vi "CIS.vi"(2 "Run uninterrupted?":bool, 3 "Device Category IN:":string(combo)="ATLAS18SS" caption="Device Category:", 4 "Batch No.:":string, 5 "Sensor Serial No.:":string, 6 "DB Serial No.:":string) -> (0 "Done!":bool)   [LabVIEW 2019]
doc: "Performs Cis measurements according to ATLAS ITk Quality Control Specifications."
uses:
  general_VIs/globals/QC_MeasurementSetup.vi
  general_VIs/globals/QC_RunInformation.vi
  InstrControl/InstrumentSetup.vi
  InstrControl/Switching/Switching.lvclass
  InstrControl/SupplyControl/SupplyControl.lvclass
  InstrControl/LCRControl/LCRControl.lvclass
  InstrControl/ArduinoControl/ArduinoControl.lvclass
  <vilib>/Analysis/NI_AALBase.lvlib
  InstrControl/InstrControl.lvclass
panel:
  out "Tab Control 2":enum32{"Cis Setup", "Cis Scan"}(tab)
  in  "Current Limit [µA]":dbl=1000.0 min=0.0001 format="%.3f"
  in  "Cis @300V limit [pF/cm]":dbl=1.0
  in  "step interval [s] IN":i32=5 caption="step interval [s]"
  in  "step [V] IN":dbl=10.0 caption="step [V]" format="%.1f"
  in  "Final volts [V] IN":dbl=-500.0 caption="Final volts [V]"
  in  "Initial volts [V] IN":dbl caption="Initial volts [V]"
  in  "Frequency [Hz] Setup":i32=500 caption="Frequency [Hz]" format="%#.3p"
  in  "Measurement Configurations":bool
  in  "Continue":bool
  in  "Quit":bool
  in  "Software current limit?":bool
  out "Capacitance":dbl[](array[numeric]) caption="Cap [pF]"
  out "Volts":dbl[](array[numeric]) caption="Volts [V]"
  out "Resistance":dbl[](array[numeric]) caption="Res [kOhm]"
  out "step interval [s]":u32=5
  out "step [V]":dbl=10.0 format="%.1f"
  out "Final volts [V]":dbl=-700.0 format="%.1f"
  out "Initial volts [V]":dbl format="%.1f"
  out "Frequency [Hz]":i32=100000 format="%#.3p"
  out "RH":dbl[](array[numeric]) caption="RH [%]" format="%#.2f"
  out "Temp.":dbl[](array[numeric]) caption="Temp. [°C]" format="%#.2f"
  out "Cgraph":cluster{"Initial volts":dbl, dbl, dbl[]}(graph)
  in  "Scales":T1(ring)
  in  "Cscale":enum16{"1/C^2 [1/nF^2]", "nF", "pF"}(ring)=enum."pF"
  out "positive ramp?":bool
  out "Tab Control":enum32{"Cis Setup", "Cis Scan"}(tab)
  in  "Switching":string(combo)="Pickering Matrix"
  in  "LCR Meter":string(combo)="WayneKerr 6440B"
  in  "Cis Supply":string(combo)="Keithley 2410"
  in  "Temperature":enum16{"Read Arduino", "Enter manually"}(ring)
  in  "User:":string(combo)="Christoph"
  in  "Hardware Configurations":bool
  in  "Manufacturer:":string(combo)="Hamamatsu"
  in  "abort":bool
  out "Device Category:":string
  out "DB Serial No.:":string
  out "Current Volts:":dbl format="%.2f"
  in  "quit (no save)":bool
  in  "Quit & Save":bool
  out "Bias On/Off:":bool
  out "STATUS 1":string
  out "Initiated:":string
  out "Sensor No.:":string
  out "No of steps":u32
  out "Current reading No.":u32
  out "Last reading at:":string
  # "University of\nCambridge"
  # "Strip Sensor QC: inter-strip Capacitance"
  # "Vertical Scale:"
  # "Measurement Configuration"
  # "Cis Scan parameters:"
  # "Last 5 readings:"
  # "n-4"
  # "n-3"
  # "n-2"
  # "n-1"
  # "n"
  # "DUT Description"
  # "Hardware"
  # "DUT & Test Description:"
  # "Current status:"
  # "Rdg No:"
  # "out of"
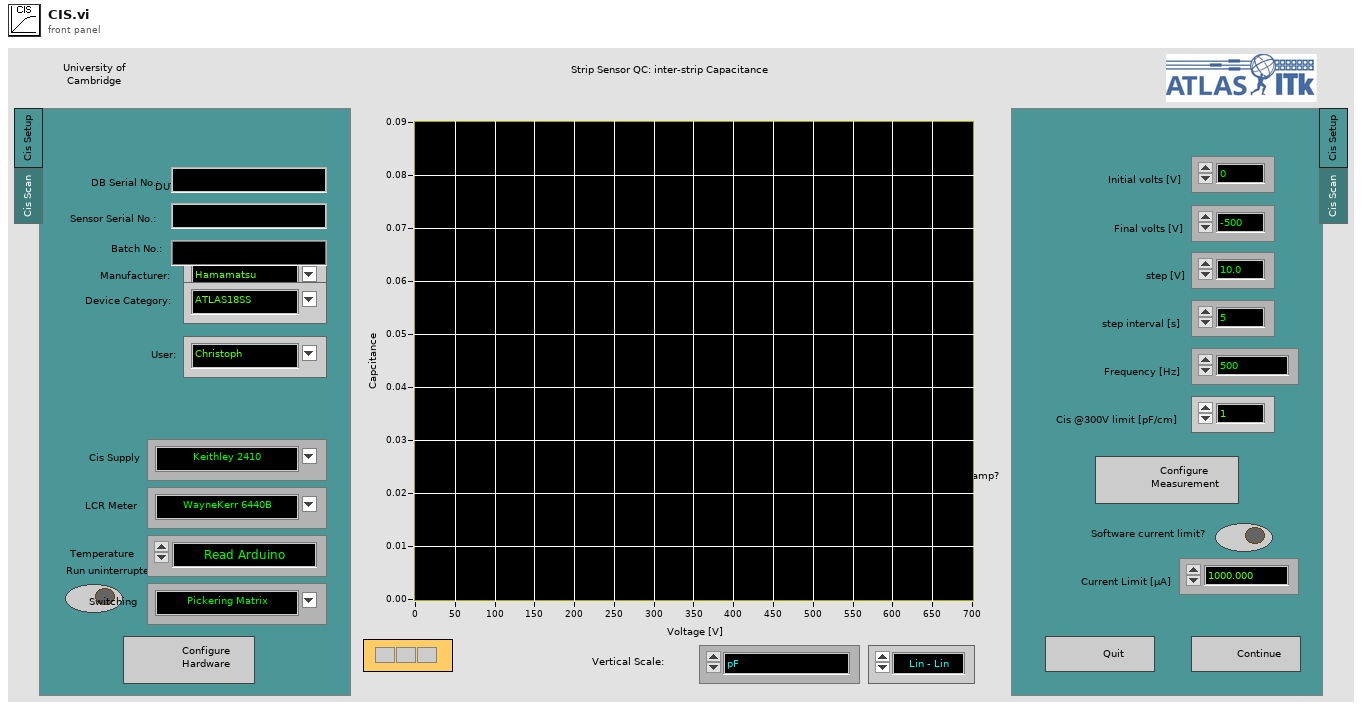
[diagram p1: front panel]
types:
  T1 = enum16{"Lin - Lin", "Log - Lin", "Lin - Log", "Log - log"}
  T2 = enum16{"Supply", "LCR", "Multimeter", "Switching"}
  T3 = enum16{"Reset", "Read Array", "Read Element", "Write Element", "Write Array", "Add Element", "Add Array"}
  T4 = enum16{"Reset", "Ground", "Striptest Bias", "Striptest SMU", "Striptest LCR", "IV", "CV", "Interstrip Cap", "Interstrip Res"}
  T5 = enum32{"IV", "CV", "Stability", "Striptest", "Cis", "Ris", "PTP"}
  T6 = cluster{"Sensor Serial No.:":string, "Wafer Serial No.:":string, "Batch:":string, "Manufacturer:":string, "Device Category:":string, "Database Serial No.:":string, "Date Initiated:":string, "Time Initiated:":string, "Test":string, "Instruments used:":string, "Probeplan used:":string, "End of Run comment:":string, "User:":string}
  T7 = cluster{"Institute":string, "Manufacturers":string[], "Devices":string[], "Serialnumbers Lookup DB":string, "Data directory":string, "Backup & screenshot directory":string, "List of known users":string[], "Measurement switch not used":bool, "Measurement Switch":string, "DUT Switch":string}
  T8 = cluster{"Supply":refnum<class "SupplyControl.lvclass">, "LCR":refnum<class "LCRControl.lvclass">, "Initial Voltage [V]":dbl, "Final Voltage [V]":dbl, "Step Size [V]":dbl, "Step Interval [s]":i32, "Number Of Steps":u32, "AC frequency [Hz]":i32, "RC Configuration":u16, "AC amplitude [V]":dbl, "Ramp down steps [V]":dbl, "Ramp down Interval [s]":i32, "Set Current Limit?":bool, "Current Limit [µA]":dbl, "Temperature Readout":enum16{"Read Arduino", "Enter manually"}, "Arduino":refnum<class "ArduinoControl.lvclass">, "Supply Name":string, "LCR Name":string, "C_is Limit [pF/cm]":dbl, "Switching":refnum<class "Switching.lvclass">, "Matrix used?":bool, "Matrix X Channels":cluster{"Bias Supply / SMU LO":i32, "Bias Supply / SMU HI":i32, "CV Box LO":i32, "CV Box HI":i32, "CV Box LO IN":i32, "CV Box HI IN":i32, "Volt meter LO":i32, "Volt meter HI":i32, "Mux1 C1":i32, "Mux1 C2":i32, "Mux2 C1":i32, "Mux2 C2":i32}}
  T9 = cluster{"VISA address":refnum<visa-resource-name>, "T sensor":enum16{"SHT", "DS"}, "Arduino":refnum<class "ArduinoControl.lvclass">}
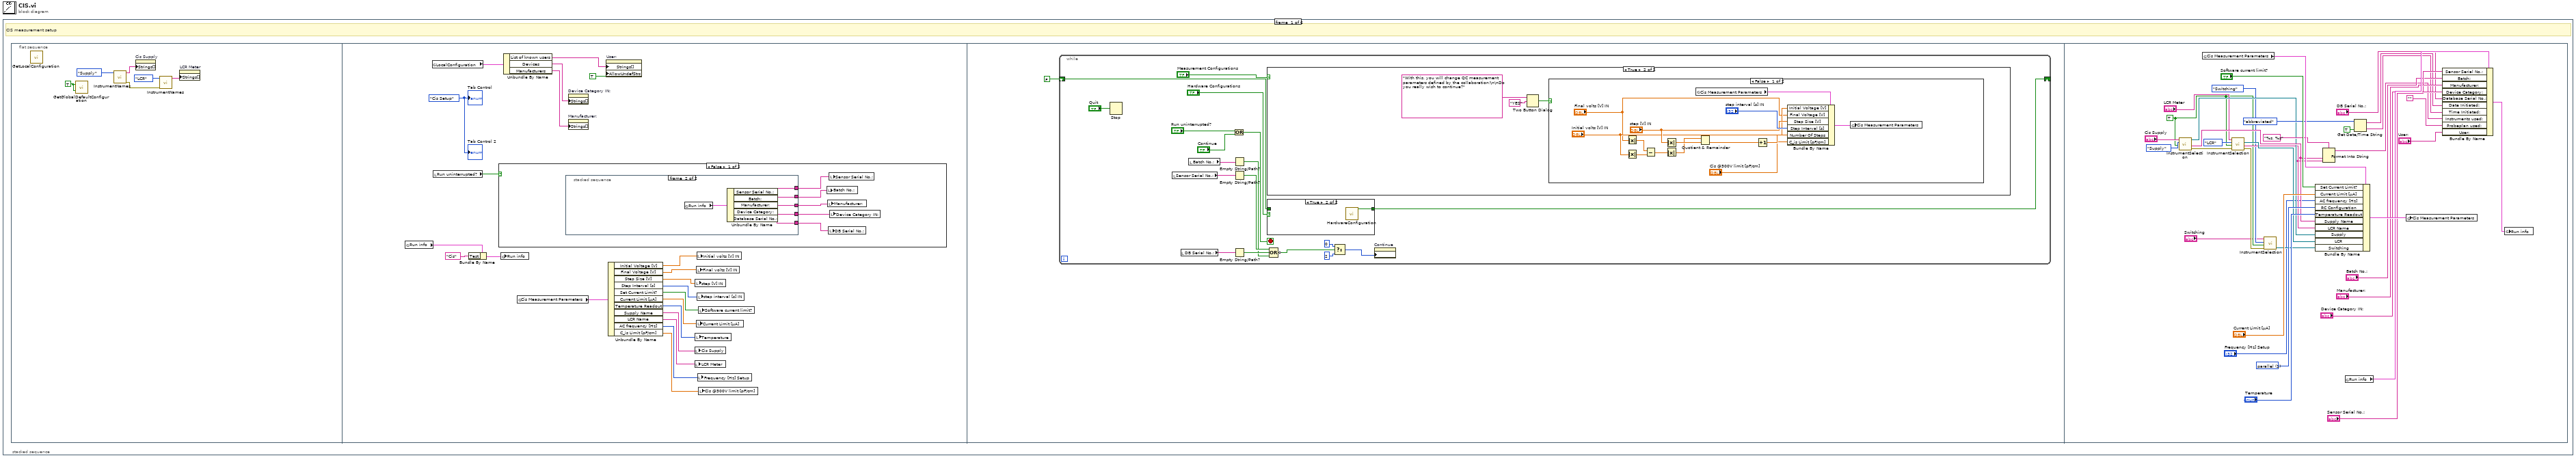
[diagram p0: block diagram]
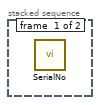
[diagram p2: hidden frame]
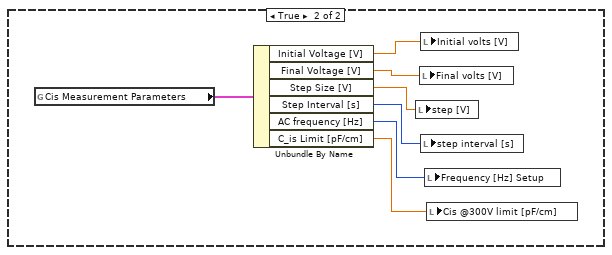
[diagram p6: hidden frame]
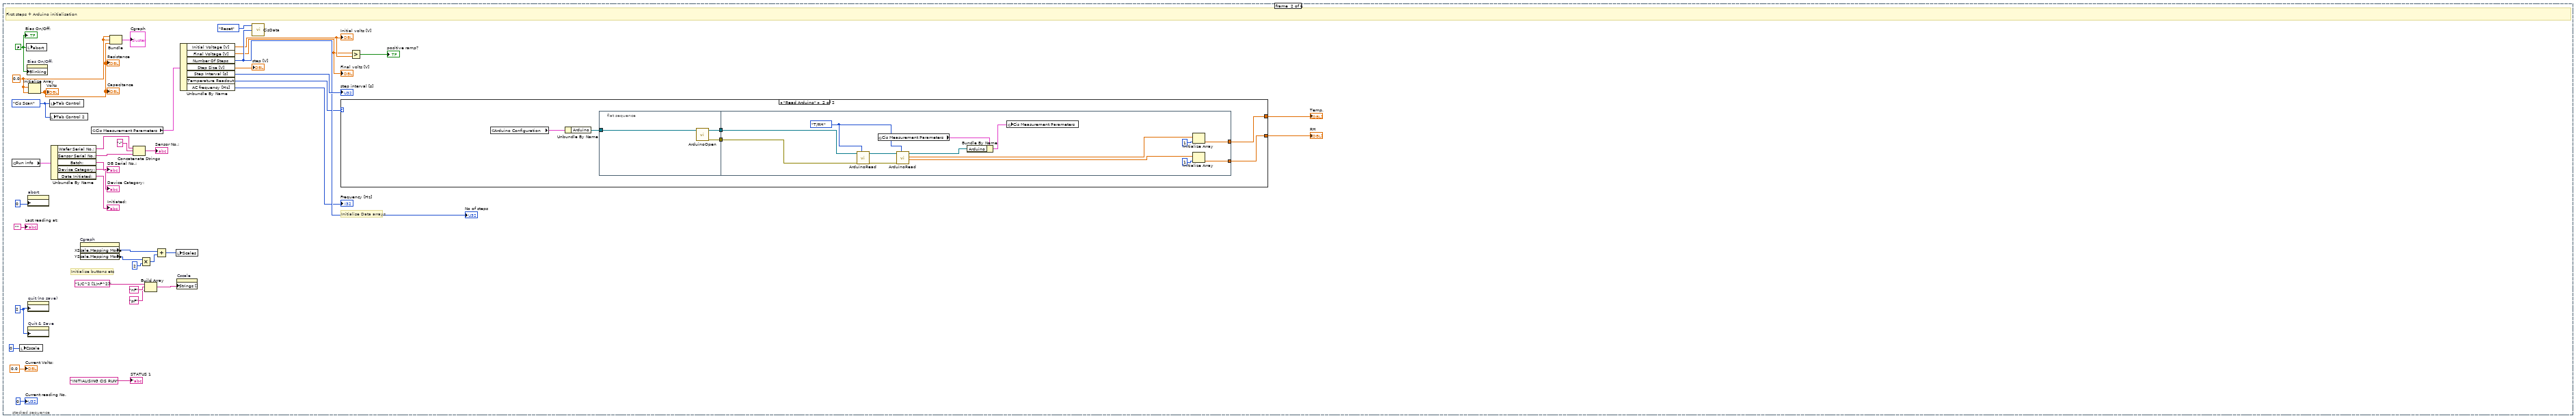
[diagram p7: hidden frame]
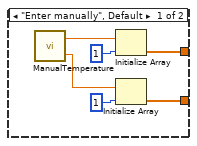
[diagram p8: hidden frame]
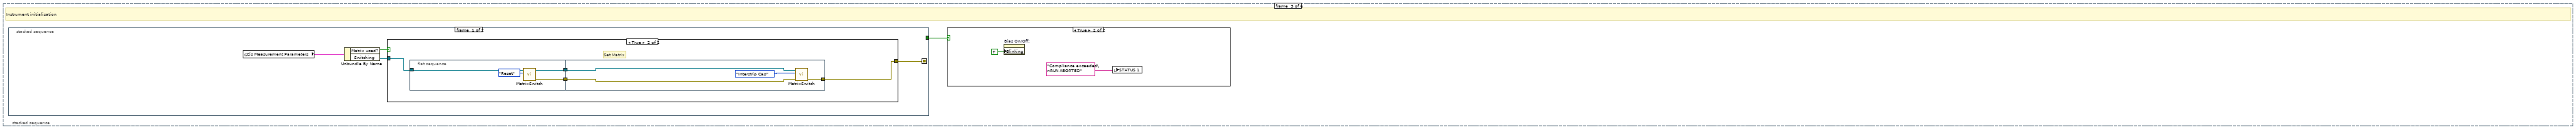
[diagram p9: hidden frame]
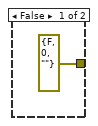
[diagram p10: hidden frame]
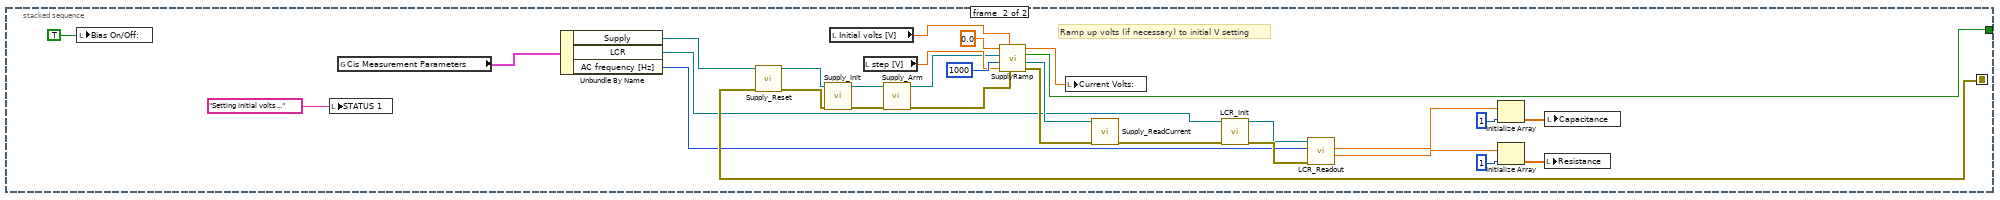
[diagram p11: hidden frame]
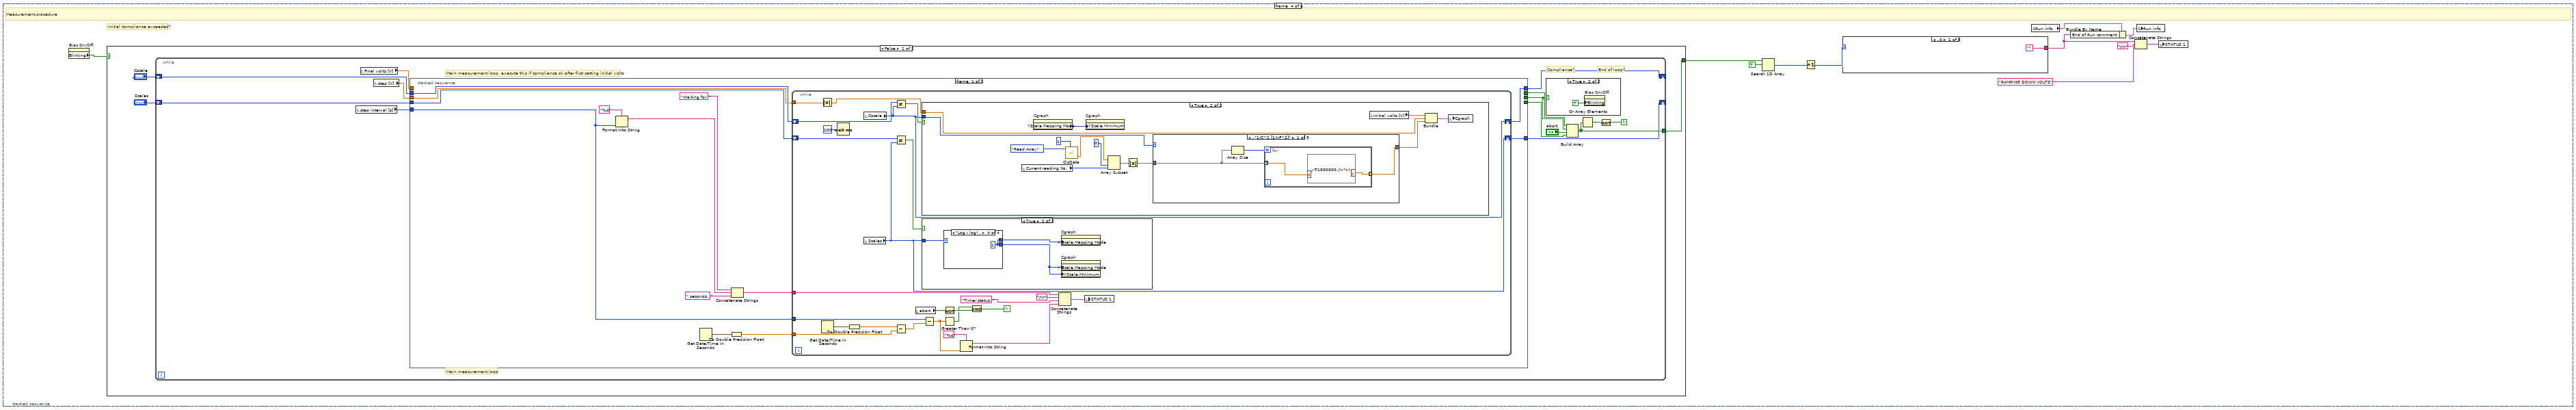
[diagram p13: hidden frame]
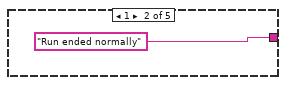
[diagram p14: hidden frame]
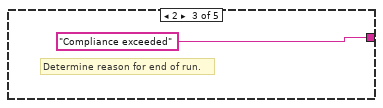
[diagram p15: hidden frame]
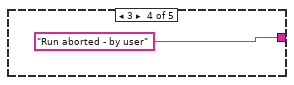
[diagram p16: hidden frame]
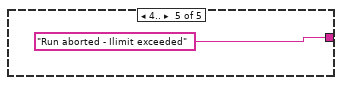
[diagram p17: hidden frame]
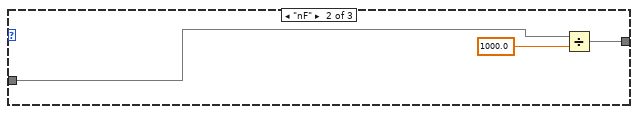
[diagram p19: hidden frame]
diagram:
  n1 = stacked-sequence {
    frame #0 {
      # "CIS measurement setup"
      n2 = flat-sequence {
        frame #0 {
          w6 = TRUE
          n3 = call "GetLocalConfiguration.vi"() -> ()  [unwired: 3 in, 1 out]
          n4 = call "GetGlobalDefaultConfiguration.vi"("DO NOT override instruments"=w6, "Read defaults?"=w6) -> ()  [unwired: 1 in, 1 out]
          n5 = call "InstrumentNames.vi"("Instrument type"=T2."Supply") -> ("error out"=w3:errorcluster, "Instrument names"=w1:string[])  [unwired: 9 in]
          n6 = property on="Cis Supply" class="CmbBox"("Strings[]"=w1) -> ()  [unwired: 2 in, 2 out]
          n7 = call "InstrumentNames.vi"("error in (no error)"=w3, "Instrument type"=T2."LCR") -> ("Instrument names"=w2:string[])  [unwired: 8 in, 1 out]
          n8 = property on="LCR Meter" class="CmbBox"("Strings[]"=w2) -> ()  [unwired: 2 in, 2 out]
        }
        frame #1 {
          w15 = enum32{"Cis Setup", "Cis Scan"}."Cis Setup" ("Tab Control")
          n9 = global read "QC_RunInformation.vi" "Run info"() -> (w16:T6)
          n10 = global read "QC_RunInformation.vi" "LocalConfiguration"() -> (w23:T7)
          n11 = local read "Run uninterrupted?"() -> (w14:bool)
          n12 = Bundle By Name(cluster=w16, "Test"="Cis") -> (w18:T6)
          n13 = case shown="False" w14 {
            frame False {
              n14 = stacked-sequence {
                tunnel: [_ w39] -> w33
                tunnel: [_ w38] -> w32
                tunnel: [_ w37] -> w31
                tunnel: [_ w36] -> w29
                tunnel: [_ w34] -> w30
                frame #0 {
                  n15 = call "SerialNo.vi"() -> ()  [unwired: 5 in, 1 out]
                }
                frame #1 {
                  n16 = global read "QC_RunInformation.vi" "Run info"() -> (w35:T6)
                  n17 = Unbundle By Name(w35) -> ("Sensor Serial No.:"=w39:string, "Batch:"=w38:string, "Manufacturer:"=w37:string, "Device Category:"=w36:string, "Database Serial No.:"=w34:string)
                }
              }
              n18 = local write "Batch No.:"(w32) -> ()
              n19 = local write "Manufacturer:"(w31) -> ()
              n20 = local write "DB Serial No.:"(w30) -> ()
              n21 = local write "Sensor Serial No.:"(w33) -> ()
              n22 = local write "Device Category IN:"(w29) -> ()
            }
            frame True {
            }
          }
          n23 = global write "QC_RunInformation.vi" "Run info"(w18) -> ()
          n24 = Unbundle By Name(w23) -> ("List of known users"=w22:string[], "Devices"=w7:string[], "Manufacturers"=w8:string[])
          n25 = global read "QC_MeasurementSetup.vi" "Cis Measurement Parameters"() -> (w26:T8)
          n26 = property on="Device Category IN:" class="CmbBox"("Strings[]"=w7) -> ()  [unwired: 2 in, 2 out]
          n27 = property on="Manufacturer:" class="CmbBox"("Strings[]"=w8) -> ()  [unwired: 2 in, 2 out]
          n28 = property on="User:" class="CmbBox"("Strings[]"=w22, "AllowUndefStrs"=TRUE) -> ()  [unwired: 2 in, 2 out]
          n29 = Unbundle By Name(w26) -> ("Initial Voltage [V]"=w11:dbl, "Final Voltage [V]"=w12:dbl, "Step Size [V]"=w10:dbl, "Step Interval [s]"=w13:i32, "Set Current Limit?"=w25:bool, "Current Limit [µA]"=w24:dbl, "Temperature Readout"=w28:enum16{"Read Arduino", "Enter manually"}, "Supply Name"=w27:string, "LCR Name"=w20:string, "AC frequency [Hz]"=w19:i32, "C_is Limit [pF/cm]"=w9:dbl)
          n30 = local write "Cis Supply"(w27) -> ()
          n31 = local write "LCR Meter"(w20) -> ()
          n32 = local write "step [V] IN"(w10) -> ()
          n33 = local write "Temperature"(w28) -> ()
          n34 = local write "Final volts [V] IN"(w12) -> ()
          n35 = local write "Current Limit [µA]"(w24) -> ()
          n36 = local write "Initial volts [V] IN"(w11) -> ()
          n37 = local write "step interval [s] IN"(w13) -> ()
          n38 = local write "Frequency [Hz] Setup"(w19) -> ()
          n39 = local write "Software current limit?"(w25) -> ()
          n40 = local write "Cis @300V limit [pF/cm]"(w9) -> ()
          "Tab Control" <- w15
          "Tab Control 2" <- w15
        }
        frame #2 {
          n41 = while {
            shift-right: [w41] -> _
            shift-left: FALSE -> [w42]
            stop <- w45 stop-if-true
            n42 = Stop(stop? (T)="Quit") -> ()
            n43 = local read "Sensor Serial No.:"() -> (w57:string)
            n44 = local read "DB Serial No.:"() -> (w56:string)
            n45 = local read "Batch No.:"() -> (w49:string)
            n46 = Or(x="Run uninterrupted?", y="Continue") -> (x .or. y?=w45:bool)
            n47 = Empty String/Path?(string/path=w49) -> (empty?=w48:bool)
            n48 = Empty String/Path?(string/path=w57) -> (empty?=w54:bool)
            n49 = Empty String/Path?(string/path=w56) -> (empty?=w55:bool)
            n50 = case shown="True" "Measurement Configurations" {
              frame False {
              }
              frame True {
                n51 = Two Button Dialog(message="With this, you will change QC measurement parameters defined by the collaboration!\n\nDo you really wish to continue?", 2:"YES") -> (T button?=w61:bool)  [unwired: 1 in]
                n52 = case shown="False" w61 {
                  frame False {
                    n53 = Absolute Value(x="Final volts [V] IN") -> (abs(x)=w74:dbl)
                    n54 = Absolute Value(x="Initial volts [V] IN") -> (abs(x)=w73:dbl)
                    n55 = Subtract(x=w74, y=w73) -> (x-y=w71:dbl)
                    n56 = Absolute Value(x="step [V] IN") -> (abs(x)=w72:dbl)
                    n57 = Absolute Value(x=w71) -> (abs(x)=w67:dbl)
                    n58 = global read "QC_MeasurementSetup.vi" "Cis Measurement Parameters"() -> (w76:T8)
                    n59 = Quotient & Remainder(x=w67, y=w72) -> (floor(x/y)=w75:dbl)  [unwired: 1 out]
                    n60 = Increment(x=w75) -> (x+1=w70:dbl)
                    n61 = Bundle By Name(cluster=w76, "Initial Voltage [V]"="Initial volts [V] IN", "Final Voltage [V]"="Final volts [V] IN", "Step Size [V]"="step [V] IN", "Step Interval [s]"="step interval [s] IN", "Number Of Steps"=w70, "C_is Limit [pF/cm]"="Cis @300V limit [pF/cm]") -> (w77:T8)
                    n62 = global write "QC_MeasurementSetup.vi" "Cis Measurement Parameters"(w77) -> ()
                  }
                  frame True {
                    n63 = global read "QC_MeasurementSetup.vi" "Cis Measurement Parameters"() -> (w84:T8)
                    n64 = Unbundle By Name(w84) -> ("Initial Voltage [V]"=w82:dbl, "Final Voltage [V]"=w83:dbl, "Step Size [V]"=w81:dbl, "Step Interval [s]"=w80:i32, "AC frequency [Hz]"=w79:i32, "C_is Limit [pF/cm]"=w78:dbl)
                    n65 = local write "step [V]"(w81) -> ()
                    n66 = local write "Final volts [V]"(w83) -> ()
                    n67 = local write "Initial volts [V]"(w82) -> ()
                    n68 = local write "step interval [s]"(w80) -> ()
                    n69 = local write "Frequency [Hz] Setup"(w79) -> ()
                    n70 = local write "Cis @300V limit [pF/cm]"(w78) -> ()
                  }
                }
              }
            }
            n71 = case shown="True" "Hardware Configurations" {
              tunnel: [w59 w60] -> w41
              tunnel: w42 -> [w59 _]
              frame False {
              }
              frame True {
                n72 = call "HardwareConfiguration.vi"() -> ("configured?"=w60:bool)  [unwired: 11 in]
              }
            }
            n73 = Compound Arithmetic op=OR(w54, w55, w48) -> (invert w53:bool)
            n74 = Select(t=0, s=w53, f=2) -> (s? t:f=w50:i32)
            n75 = property on="Continue" class="Bool"("DisabledEnum"=w50) -> ()  [unwired: 2 in, 2 out]
          }
        }
        frame #3 {
          w91 = TRUE
          w106 = u16 1 items=["serial", "parallel"] ("RC Configuration")
          n76 = call "InstrumentSelection.vi"("Verify GPIB address"=w91, "Instrument type"=T2."Supply", "Instrument name IN"="Cis Supply") -> ("error out"=w96:errorcluster, "Instrument name OUT"=w101:string, "Supply"=w100:refnum<class "SupplyControl.lvclass">)  [unwired: 3 in, 3 out]
          n77 = global read "QC_MeasurementSetup.vi" "Cis Measurement Parameters"() -> (w119:T8)
          n78 = call "InstrumentSelection.vi"("error in (no error)"=w96, "Verify GPIB address"=w91, "Instrument type"=T2."LCR", "Instrument name IN"="LCR Meter") -> ("error out"=w92:errorcluster, "Instrument name OUT"=w97:string, "LCR"=w99:refnum<class "LCRControl.lvclass">)  [unwired: 2 in, 3 out]
          n79 = call "InstrumentSelection.vi"("error in (no error)"=w92, "Verify GPIB address"=w91, "Instrument type"=T2."Switching", "Instrument name IN"="Switching") -> ("Switching"=w90:refnum<class "Switching.lvclass">)  [unwired: 2 in, 5 out]
          n80 = Bundle By Name(cluster=w119, "Set Current Limit?"="Software current limit?", "Current Limit [µA]"="Current Limit [µA]", "AC frequency [Hz]"="Frequency [Hz] Setup", "RC Configuration"=w106, "Temperature Readout"="Temperature", "Supply Name"=w101, "LCR Name"=w97, "Supply"=w100, "LCR"=w99, "Switching"=w90) -> (w120:T8)
          n81 = Format Into String(format string="%s, %s", w101, w97) -> (resulting string=w103:string)  [unwired: 2 in, 1 out]
          n82 = global read "QC_RunInformation.vi" "Run info"() -> (w114:T6)
          n83 = Get Date/Time String(date format (0)=enum16{"short", "long", "abbreviated"}."abbreviated", want seconds? (F)=TRUE) -> (date string=w87:string, time string=w86:string)  [unwired: 1 in]
          n84 = global write "QC_MeasurementSetup.vi" "Cis Measurement Parameters"(w120) -> ()
          n85 = Bundle By Name(cluster=w114, "Sensor Serial No.:"="Sensor Serial No.:", "Batch:"="Batch No.:", "Manufacturer:"="Manufacturer:", "Device Category:"="Device Category IN:", "Database Serial No.:"="DB Serial No.:", "Date Initiated:"=w87, "Time Initiated:"=w86, "Instruments used:"=w103, "Probeplan used:"="", "User:"="User:") -> (w113:T6)
          n86 = global write "QC_RunInformation.vi" "Run info"(w113) -> ()
        }
      }
    }
    frame #1 {
      w121 = enum32{"Cis Setup", "Cis Scan"}."Cis Scan" ("Tab Control")
      w143 = 2
      w150 = 0.0
      w142 = FALSE ("Visible")
      # "Initialise buttons etc"
      # "Initialise Data arrays"
      # "First steps + Arduino initialisation"
      n87 = global read "QC_RunInformation.vi" "Run info"() -> (w160:T6)
      n88 = local write "Cscale"(u16 0 ("Scale")) -> ()
      n89 = local write "abort"(w142) -> ()
      n90 = property on="Bias On/Off:" class="Bool (strict)"("Blinking"=w142) -> ()  [unwired: 2 in, 2 out]
      n91 = property on="abort" class="Bool (strict)"("DisabledEnum"=0) -> ()  [unwired: 2 in, 2 out]
      n92 = property on="quit (no save)" class="Bool"("DisabledEnum"=w143) -> ()  [unwired: 2 in, 2 out]
      n93 = property on="Quit & Save" class="Bool"("DisabledEnum"=w143) -> ()  [unwired: 2 in, 2 out]
      n94 = Initialize Array(w150, w150) -> (w123:dbl[])
      "Volts" <- w123
      "Capacitance" <- w123
      "Resistance" <- w123
      n95 = local write "Tab Control"(w121) -> ()
      n96 = local write "Tab Control 2"(w121) -> ()
      n97 = Unbundle By Name(w160) -> ("Wafer Serial No.:"=w129:string, "Sensor Serial No.:"=w128:string, "Batch:"=→"DB Serial No.:":string, "Device Category:"=→"Device Category:":string, "Date Initiated:"=→"Initiated:":string)
      n98 = property on="Cgraph" class="WFGraph (strict)"() -> ("XScale.Mapping Mode"=w135:u8, "YScale.Mapping Mode"=w134:u8)  [unwired: 2 in, 2 out]
      n99 = global read "QC_MeasurementSetup.vi" "Cis Measurement Parameters"() -> (w131:T8)
      n100 = Bundle(w150, w150, w123) -> (→"Cgraph":cluster{dbl, dbl, dbl[]})  [unwired: 1 in]
      n101 = Concatenate Strings(w129, "-", w128) -> (→"Sensor No.:":string)
      n102 = Multiply(x=w134, y=2) -> (x*y=w137:i32)
      n103 = Build Array("1/C^2 [1/nF^2]", "nF", "pF") -> (w157:string[])
      n104 = Add(x=w135, y=w137) -> (x+y=w133:i32)
      n105 = local write "Scales"(w133) -> ()
      n106 = property on="Cscale" class="Enum (strict)"("Strings []"=w157) -> ()  [unwired: 2 in, 2 out]
      n107 = Unbundle By Name(w131) -> ("Initial Voltage [V]"=w141:dbl, "Final Voltage [V]"=w140:dbl, "Number Of Steps"=w151:u32, "Step Size [V]"=→"step [V]":dbl, "Step Interval [s]"=→"step interval [s]":i32, "Temperature Readout"=w144:enum16{"Read Arduino", "Enter manually"}, "AC frequency [Hz]"=→"Frequency [Hz]":i32)
      "No of steps" <- w151
      "Initial volts [V]" <- w141
      "Final volts [V]" <- w140
      n108 = call "CisData.vi"("Action"=T3."Reset", "Array Size / Index"=w151) -> ()  [unwired: 3 in, 2 out]
      n109 = case shown="\"Read Arduino\"" w144 {
        tunnel: [w166 w173] -> w147
        tunnel: [w163 w172] -> w132
        frame "Enter manually", Default {
          n110 = call "ManualTemperature.vi"() -> ("Humidity [%] out"=w162:dbl, "Temperature [°C] out"=w167:dbl)
          n111 = Initialize Array(w167, 1) -> (w166:dbl[])
          n112 = Initialize Array(w162, 1) -> (w163:dbl[])
        }
        frame "Read Arduino" {
          n113 = global read "InstrumentSetup.vi" "Arduino Configuration"() -> (w169:T9)
          n114 = Unbundle By Name(w169) -> ("Arduino"=w168:refnum<class "ArduinoControl.lvclass">)
          n115 = flat-sequence {
            tunnel: [w174] -> w171
            tunnel: [w176] -> w170
            tunnel: w168 -> [w175]
            tunnel: [w190] -> w173
            tunnel: [w187] -> w172
            tunnel: w171 -> [w179]
            tunnel: w170 -> [w180]
            frame #0 {
              n116 = call "ArduinoOpen.vi"("ArduinoControl in"=w175) -> ("error out"=w176:errorcluster, "ArduinoControl out"=w174:refnum<class "ArduinoControl.lvclass">)  [unwired: 9 in]
            }
            frame #1 {
              w181 = enum16{"T/RH", "Interlock", "Edgesense"}."T/RH" ("Arduino function")
              n117 = call "ArduinoRead.vi"("Arduino function"=w181, "error in (no error)"=w180, "ArduinoControl in"=w179) -> ("error out"=w177:errorcluster, "ArduinoControl out"=w178:refnum<class "ArduinoControl.lvclass">)  [unwired: 3 in, 4 out]
              n118 = global read "QC_MeasurementSetup.vi" "Cis Measurement Parameters"() -> (w183:T8)
              n119 = call "ArduinoRead.vi"("Arduino function"=w181, "error in (no error)"=w177, "ArduinoControl in"=w178) -> ("rel. Humidity [%]"=w185:dbl, "Temperature [°C]"=w186:dbl, "ArduinoControl out"=w184:refnum<class "ArduinoControl.lvclass">)  [unwired: 3 in, 3 out]
              n120 = Bundle By Name(cluster=w183, "Arduino"=w184) -> (w182:T8)
              n121 = global write "QC_MeasurementSetup.vi" "Cis Measurement Parameters"(w182) -> ()
              n122 = Initialize Array(w186, 1) -> (w190:dbl[])
              n123 = Initialize Array(w185, 1) -> (w187:dbl[])
            }
          }
        }
      }
      "Temp." <- w147
      "RH" <- w132
      n124 = Greater?(x=w140, y=w141) -> (0:→"positive ramp?":bool)
      "STATUS 1" <- "INITIALISING CIS RUN"
      "Bias On/Off:" <- w142
      "Last reading at:" <- ""
      "Current reading No." <- u32 0 ("Current reading No.")
      "Current Volts:" <- 0.0 ("Current Volts:")
    }
    frame #2 {
      # "Instrument initialisation"
      n125 = stacked-sequence {
        seq-local: [w193 _] -> [_ w212]
        tunnel: [_ w213] -> w191
        frame #0 {
          n126 = global read "QC_MeasurementSetup.vi" "Cis Measurement Parameters"() -> (w192:T8)
          n127 = Unbundle By Name(w192) -> ("Matrix used?"=w195:bool, "Switching"=w194:refnum<class "Switching.lvclass">)
          n128 = case shown="True" w195 {
            tunnel: w194 -> [_ w197]
            tunnel: [errorcluster {"status"=FALSE, "code"=0, "source"=""} ("error constant") w198] -> w193
            frame False {
            }
            frame True {
              # "Set Matrix"
              n129 = flat-sequence {
                tunnel: [w204] -> w200
                tunnel: [w203] -> w199
                tunnel: w197 -> [w202]
                tunnel: w200 -> [w208]
                tunnel: w199 -> [w207]
                tunnel: [w206] -> w198
                frame #0 {
                  n130 = call-dynamic "MatrixSwitch.vi"("Action"=T4."Reset", "Switching in"=w202) -> ("error out"=w204:errorcluster, "Switching out"=w203:refnum<class "Switching.lvclass">)  [unwired: 7 in, 1 out]
                }
                frame #1 {
                  n131 = call-dynamic "MatrixSwitch.vi"("error in (no error)"=w208, "Action"=T4."Interstrip Cap", "Switching in"=w207) -> ("error out"=w206:errorcluster)  [unwired: 6 in, 2 out]
                }
              }
            }
          }
        }
        frame #1 {
          # "Ramp up volts (if necessary) to initial V setting"
          n132 = local write "Bias On/Off:"(TRUE ("Compliance?")) -> ()
          n133 = local write "STATUS 1"("Setting initial volts..." ("STATUS 1")) -> ()
          n134 = global read "QC_MeasurementSetup.vi" "Cis Measurement Parameters"() -> (w234:T8)
          n135 = Unbundle By Name(w234) -> ("Supply"=w231:refnum<class "SupplyControl.lvclass">, "LCR"=w210:refnum<class "LCRControl.lvclass">, "AC frequency [Hz]"=w209:i32)
          n136 = call-dynamic "Supply_Reset.vi"("error in (no error)"=w212, "SupplyControl in"=w231) -> ("error out"=w236:errorcluster, "SupplyControl out"=w238:refnum<class "SupplyControl.lvclass">)  [unwired: 8 in]
          n137 = call-dynamic "Supply_Init.vi"("error in (no error)"=w236, "SupplyControl in"=w238) -> ("error out"=w235:errorcluster, "SupplyControl out"=w237:refnum<class "SupplyControl.lvclass">)  [unwired: 8 in]
          n138 = local read "Initial volts [V]"() -> (w216:dbl)
          n139 = local read "step [V]"() -> (w217:dbl)
          n140 = call-dynamic "Supply_Arm.vi"("error in (no error)"=w235, "SupplyControl in"=w237) -> ("error out"=w214:errorcluster, "SupplyControl out"=w215:refnum<class "SupplyControl.lvclass">)  [unwired: 8 in]
          n141 = call "SupplyRamp.vi"("error in"=w214, "Requested Voltage"=w216, "Step Size"=w217, "Step Delay"=1000, "Supply IN"=w215, "Starting Voltage"=0.0) -> ("error out"=w230:errorcluster, "Supply OUT"=w211:refnum<class "SupplyControl.lvclass">, "Compliance exceeded"=w213:bool, "Current Voltage"=w220:dbl)  [unwired: 2 in]
          n142 = local write "Current Volts:"(w220) -> ()
          n143 = call-dynamic "Supply_ReadCurrent.vi"("error in (no error)"=w230, "SupplyControl in"=w211) -> ("error out"=w227:errorcluster)  [unwired: 7 in, 2 out]
          n144 = call-dynamic "LCR_Init.vi"("error in (no error)"=w227, "LCRControl in"=w210) -> ("error out"=w229:errorcluster, "LCRControl out"=w228:refnum<class "LCRControl.lvclass">)  [unwired: 8 in]
          n145 = call-dynamic "LCR_Readout.vi"("error in (no error)"=w229, "Frequency in Hz"=w209, "LCRControl in"=w228) -> ("Resistance in Ohm"=w225:dbl, "Capacitance in pF"=w226:dbl)  [unwired: 5 in, 2 out]
          n146 = Initialize Array(w226, 1) -> (w221:dbl[])
          n147 = Initialize Array(w225, 1) -> (w224:dbl[])
          n148 = local write "Resistance"(w224) -> ()
          n149 = local write "Capacitance"(w221) -> ()
        }
      }
      n150 = case shown="True" w191 {
        frame False {
        }
        frame True {
          n151 = property on="Bias On/Off:" class="Bool (strict)"("Blinking"=TRUE) -> ()  [unwired: 2 in, 2 out]
          n152 = local write "STATUS 1"("Compliance exceeded\nRUN ABORTED") -> ()
        }
      }
    }
    frame #3 {
      # "Initial compliance exceeded?"
      # "Measurement procedure"
      n153 = property on="Bias On/Off:" class="Bool (strict)"() -> ("Blinking"=w251:bool)  [unwired: 2 in, 2 out]
      n154 = case shown="False" w251 {
        tunnel: [w259 w506] -> w250
        frame False {
          n155 = while {
            shift-left: "Cscale" -> [w269]
            shift-right: [w268] -> _
            shift-left: "Scales" -> [w270]
            shift-right: [w271] -> _
            tunnel: [w267] -> w259
            stop <- w272 continue-if-true
            # "Main measurement loop"
            # "End of loop?"
            # "Compliance?"
            # "Main measurement loop. execute this if compliance ok after first setting initial volts"
            n156 = local read "step interval [s]"() -> (w264:u32)
            n157 = local read "Final volts [V]"() -> (w265:dbl)
            n158 = local read "step [V]"() -> (w266:dbl)
            n159 = stacked-sequence {
              tunnel: [w286 _] -> w271
              tunnel: w266 -> [w283 w349]
              tunnel: [_ w348] -> w261
              tunnel: w265 -> [_ w347]
              tunnel: w264 -> [w274 w346]
              tunnel: [_ w345] -> w263
              tunnel: w270 -> [w285 _]
              tunnel: w269 -> [w284 _]
              tunnel: [w282 _] -> w268
              tunnel: [_ w343] -> w262
              frame #0 {
                n160 = Format Into String(format string="%d", w274) -> (resulting string=w279:string)  [unwired: 2 in, 1 out]
                n161 = Get Date/Time In Seconds() -> (seconds since 1Jan1904=w276:timestamp)
                n162 = To Double Precision Float(number=w276) -> (double precision float=w277:dbl)
                n163 = Concatenate Strings("Waiting for  ", w279, " seconds...") -> (w275:string)
                n164 = while {
                  tunnel: w283 -> [w295]
                  shift-left: w284 -> [w299]
                  shift-right: [w292] -> w282
                  shift-left: w285 -> [w300]
                  shift-right: [w301] -> w286
                  tunnel: w275 -> [w293]
                  tunnel: w274 -> [w305]
                  tunnel: w277 -> [w306]
                  stop <- w307 continue-if-true
                  n165 = Absolute Value(x=w295) -> (abs(x)=w294:dbl)
                  n166 = Get Date/Time In Seconds() -> (seconds since 1Jan1904=w291:timestamp)
                  n167 = Wait (ms)(milliseconds to wait=u32 100) -> ()  [unwired: 1 out]
                  n168 = To Double Precision Float(number=w291) -> (double precision float=w311:dbl)
                  n169 = local read "Cscale"() -> (w292:enum16{"1/C^2 [1/nF^2]", "nF", "pF"})
                  n170 = local read "Scales"() -> (w301:T1)
                  n171 = Not Equal?(x=w299, y=w292) -> (x != y?=w290:bool)
                  n172 = Not Equal?(x=w300, y=w301) -> (x != y?=w302:bool)
                  n173 = Subtract(x=w311, y=w306) -> (x-y=w288:dbl)
                  n174 = local read "abort"() -> (w304:bool)
                  n175 = case shown="True" w290 {
                    tunnel: w294 -> [_ w323]
                    tunnel: w292 -> [_ w316]
                    frame False {
                    }
                    frame True {
                      n176 = local read "Current reading No."() -> (w321:u32)
                      n177 = property on="Cgraph" class="WFGraph (strict)"() -> ("YScale.Mapping Mode"=w318:u8)  [unwired: 2 in, 2 out]
                      n178 = call "CisData.vi"("Action"=T3."Read Array", "Array No."=u32 1 ("Action")) -> ("Array OUT"=w312:dbl[])  [unwired: 3 in, 1 out]
                      n179 = property on="Cgraph" class="WFGraph (strict)"("YScale.Minimum"=w318) -> ()  [unwired: 2 in, 2 out]
                      n180 = Array Subset(array=w312, index=0, length=w321) -> (w319:dbl[])
                      n181 = Absolute Value(x=w319) -> (abs(x)=w317:dbl[])
                      n182 = case shown="..\"1/C^2 [1/nF^2]\"" w316 {
                        tunnel: [w327 w330 w333] -> w315
                        tunnel: w317 -> [w325 w332 w333]
                        frame .."1/C^2 [1/nF^2]" {
                          n183 = Array Size(array=w325) -> (size(s)=w326:i32)
                          n184 = for {
                            N: w326 -> [_]
                            tunnel: w325 -> [w329] mode=indexing
                            tunnel: [w328] -> w327 mode=indexing
                            n185 = formula code="y=1000000./(x*x);"("x"=w329) -> ("y"=w328:dbl)
                          }
                        }
                        frame "nF" {
                          n186 = Divide(x=w332, y=1000.0) -> (x/y=w330:dbl[])
                        }
                        frame "pF".. {
                        }
                      }
                      n187 = local read "Initial volts [V]"() -> (w322:dbl)
                      n188 = Bundle("Initial volts [V]"=w322, w323, w315) -> (w320:cluster{"Initial volts [V]":dbl, dbl, dbl[]})  [unwired: 1 in]
                      n189 = local write "Cgraph"(w320) -> ()
                    }
                  }
                  n190 = case shown="True" w302 {
                    tunnel: w301 -> [_ w336]
                    frame False {
                    }
                    frame True {
                      n191 = case shown="\"Log - log\".." w336 {
                        tunnel: [w337 1 0 w342] -> w335
                        tunnel: [w337 0 1 w342] -> w334
                        frame .."Lin - Lin" {
                          w337 = 0
                        }
                        frame "Log - Lin" {
                        }
                        frame "Lin - Log" {
                        }
                        frame "Log - log".. {
                          w342 = 1
                        }
                      }
                      n192 = property on="Cgraph" class="WFGraph (strict)"("X Scale.Mapping Mode"=w335) -> ()  [unwired: 2 in, 2 out]
                      n193 = property on="Cgraph" class="WFGraph (strict)"("Y Scale.Mapping Mode"=w334, "YScale.Minimum"=w334) -> ()  [unwired: 2 in, 2 out]
                    }
                  }
                  n194 = Subtract(x=w305, y=w288) -> (x-y=w287:dbl)
                  n195 = Not(x=w304) -> (.not. x?=w310:bool)
                  n196 = Greater Than 0?(x=w287) -> (x > 0?=w289:bool)
                  n197 = Format Into String(format string="%d", w287) -> (resulting string=w309:string)  [unwired: 2 in, 1 out]
                  n198 = And(x=w289, y=w310) -> (x .and. y?=w307:bool)
                  n199 = Concatenate Strings(w293, "\r\n", "Timer status: ", w309) -> (w303:string)
                  n200 = local write "STATUS 1"(w303) -> ()
                }
              }
              frame #1 {
                n201 = local read "abort"() -> (w344:bool)
                n202 = case shown="False" w344 {
                  tunnel: [w355 w503] -> w345
                  tunnel: w346 -> [w354 _]
                  tunnel: w347 -> [w353 _]
                  tunnel: [w351 w503] -> w348
                  tunnel: w349 -> [w352 _]
                  tunnel: [w350 w503] -> w343
                  frame False {
                    n203 = stacked-sequence {
                      seq-local: [w381 _ _] -> [_ w405 _]
                      seq-local: [w380 _ _] -> [_ _ w472]
                      seq-local: [w367 _ _] -> [_ _ w473]
                      tunnel: w352 -> [_ w417 w478]
                      tunnel: w353 -> [_ _ w469]
                      tunnel: [_ _ w476] -> w355
                      tunnel: [_ _ w475] -> w351
                      tunnel: w354 -> [_ _ _]
                      tunnel: [w383 _ _] -> w350
                      frame #0 {
                        w363 = T3."Write Element" ("Action")
                        # "SMU data"
                        n204 = Get Date/Time String(want seconds? (F)=TRUE) -> (time string=w382:string)  [unwired: 2 in, 1 out]
                        n205 = local write "Last reading at:"(w382) -> ()
                        n206 = local write "STATUS 1"("Reading LCR meter..." ("status")) -> ()
                        n207 = global read "QC_MeasurementSetup.vi" "Cis Measurement Parameters"() -> (w379:T8)
                        n208 = Unbundle By Name(w379) -> ("Temperature Readout"=w357:enum16{"Read Arduino", "Enter manually"}, "Arduino"=w356:refnum<class "ArduinoControl.lvclass">, "LCR"=w373:refnum<class "LCRControl.lvclass">, "AC frequency [Hz]"=w358:i32, "Supply"=w374:refnum<class "SupplyControl.lvclass">, "Set Current Limit?"=w378:bool, "Current Limit [µA]"=w376:dbl)
                        n209 = local read "Current reading No."() -> (w362:u32)
                        n210 = case shown="\"Read Arduino\"" w357 {
                          tunnel: [w390 w393] -> w360
                          tunnel: [w387 w396] -> w365
                          tunnel: w356 -> [_ w395]
                          frame "Enter manually", Default {
                            n211 = local read "Temp."() -> (w392:dbl[])
                            n212 = local read "RH"() -> (w388:dbl[])
                            n213 = Index Array(array=w392, index=0) -> (element=w390:dbl)
                            n214 = Index Array(array=w388, index=0) -> (element=w387:dbl)
                          }
                          frame "Read Arduino" {
                            n215 = call "ArduinoRead.vi"("Arduino function"=enum16{"T/RH", "Interlock", "Edgesense"}."T/RH", "ArduinoControl in"=w395) -> ("rel. Humidity [%]"=w396:dbl, "Temperature [°C]"=w393:dbl)  [unwired: 4 in, 4 out]
                          }
                        }
                        n216 = local read "Current Volts:"() -> (w366:dbl)
                        n217 = Multiply(x=w376, y=1000.0) -> (x*y=w375:dbl)
                        n218 = call-dynamic "Supply_ReadCurrent.vi"("SupplyControl in"=w374) -> ("error out"=w368:errorcluster, "Current in nA"=w384:dbl, "SupplyControl out"=w380:refnum<class "SupplyControl.lvclass">)  [unwired: 8 in]
                        n219 = case shown="True" w378 {
                          tunnel: w384 -> [_ w401]
                          tunnel: w375 -> [_ w399]
                          tunnel: [FALSE w398] -> w383
                          frame False {
                          }
                          frame True {
                            n220 = Absolute Value(x=w401) -> (abs(x)=w400:dbl)
                            n221 = Greater?(x=w400, y=w399) -> (0:w398:bool)
                          }
                        }
                        n222 = call "CisData.vi"("Action"=w363, "Array No."=0, "Array Size / Index"=w362, "Data IN"=w366) -> ()  [unwired: 1 in, 2 out]
                        n223 = call-dynamic "LCR_Readout.vi"("error in (no error)"=w368, "Frequency in Hz"=w358, "LCRControl in"=w373) -> ("error out"=w367:errorcluster, "Resistance in Ohm"=w361:dbl, "Capacitance in pF"=w359:dbl)  [unwired: 5 in, 1 out]
                        n224 = Increment(x=w362) -> (x+1=w381:u32)
                        n225 = local write "Current reading No."(w381) -> ()
                        n226 = call "CisData.vi"("Action"=w363, "Array No."=u32 1, "Array Size / Index"=w362, "Data IN"=w359) -> ()  [unwired: 1 in, 2 out]
                        n227 = call "CisData.vi"("Action"=w363, "Array No."=u32 2, "Array Size / Index"=w362, "Data IN"=w361) -> ()  [unwired: 1 in, 2 out]
                        n228 = call "CisData.vi"("Action"=w363, "Array No."=u32 3, "Array Size / Index"=w362, "Data IN"=w360) -> ()  [unwired: 1 in, 2 out]
                        n229 = call "CisData.vi"("Action"=w363, "Array No."=u32 4, "Array Size / Index"=w362, "Data IN"=w365) -> ()  [unwired: 1 in, 2 out]
                      }
                      frame #1 {
                        w414 = u32 5 ("y")
                        # "Update plots"
                        n230 = property on="Cgraph" class="WFGraph (strict)"() -> ("YScale.Mapping Mode"=w406:u8)  [unwired: 2 in, 2 out]
                        n231 = Greater?(x=w405, y=w414) -> (0:w413:bool)
                        n232 = call "CisData.vi"("Action"=T3."Read Array", "Array No."=1) -> ("Array OUT"=w403:dbl[])  [unwired: 3 in, 1 out]
                        n233 = case shown="True" w413 {
                          tunnel: w405 -> [w422 w425]
                          tunnel: w414 -> [_ w424]
                          tunnel: [w422 w424] -> w412
                          tunnel: [0 w423] -> w410
                          frame False {
                          }
                          frame True {
                            n234 = Subtract(x=w425, y=w424) -> (x-y=w423:u32)
                          }
                        }
                        n235 = property on="Cgraph" class="WFGraph (strict)"("YScale.Minimum"=w406) -> ()  [unwired: 2 in, 2 out]
                        n236 = Array Subset(array=w403, index=0, length=w405) -> (w409:dbl[])
                        n237 = local read "Cscale"() -> (w415:enum16{"1/C^2 [1/nF^2]", "nF", "pF"})
                        n238 = Absolute Value(x=w409) -> (abs(x)=w408:dbl[])
                        n239 = case shown="..\"1/C^2 [1/nF^2]\"" w415 {
                          tunnel: [w458 w461 w464] -> w420
                          tunnel: w408 -> [w456 w463 w464]
                          frame .."1/C^2 [1/nF^2]" {
                            n240 = Array Size(array=w456) -> (size(s)=w457:i32)
                            n241 = for {
                              N: w457 -> [_]
                              tunnel: w456 -> [w460] mode=indexing
                              tunnel: [w459] -> w458 mode=indexing
                              n242 = formula code="y=1000000./(x*x);"("x"=w460) -> ("y"=w459:dbl)
                            }
                          }
                          frame "nF" {
                            n243 = Divide(x=w463, y=1000.0) -> (x/y=w461:dbl[])
                          }
                          frame "pF".. {
                          }
                        }
                        n244 = for {
                          N: 5 -> [_]
                          tunnel: w412 -> [w431]
                          tunnel: w410 -> [w430]
                          tunnel: w405 -> [w429]
                          i -> [w427]
                          n245 = call "CisData.vi"("Action"=T3."Read Array", "Array No."=w427) -> ("Array OUT"=w426:dbl[])  [unwired: 3 in, 1 out]
                          n246 = case shown="2" w427 {
                            tunnel: w431 -> [w434 w438 w443 _ _]
                            tunnel: w430 -> [w435 w439 w444 _ _]
                            tunnel: w426 -> [w433 w437 w445 w449 w454]
                            tunnel: w429 -> [_ _ _ w447 w452]
                            frame ..0 {
                              n247 = Array Subset(array=w433, index=w435, length=w434) -> (w432:dbl[])
                              n248 = local write "Volts"(w432) -> ()
                            }
                            frame 1 {
                              n249 = Array Subset(array=w437, index=w439, length=w438) -> (w436:dbl[])
                              n250 = local write "Capacitance"(w436) -> ()
                            }
                            frame 2 {
                              n251 = Array Subset(array=w445, index=w444, length=w443) -> (w441:dbl[])
                              n252 = Multiply(x=w441, y=0.001) -> (x*y=w440:dbl[])
                              n253 = local write "Resistance"(w440) -> ()
                            }
                            frame 3 {
                              n254 = Decrement(x=w447) -> (x-1=w446:u32)
                              n255 = Array Subset(array=w449, index=w446, length=1) -> (w448:dbl[])
                              n256 = local write "Temp."(w448) -> ()
                            }
                            frame 4.. {
                              n257 = Decrement(x=w452) -> (x-1=w451:u32)
                              n258 = Array Subset(array=w454, index=w451, length=1) -> (w453:dbl[])
                              n259 = local write "RH"(w453) -> ()
                            }
                          }
                        }
                        n260 = local read "Initial volts [V]"() -> (w418:dbl)
                        n261 = Absolute Value(x=w417) -> (abs(x)=w416:dbl)
                        n262 = Bundle("Initial volts [V]"=w418, w416, w420) -> (w407:cluster{"Initial volts [V]":dbl, dbl, dbl[]})  [unwired: 1 in]
                        n263 = local write "Cgraph"(w407) -> ()
                      }
                      frame #2 {
                        # "Increment volts and check for end of loop"
                        n264 = local read "positive ramp?"() -> (w474:bool)
                        n265 = local read "Current Volts:"() -> (w470:dbl)
                        n266 = case shown="True" w474 {
                          tunnel: w469 -> [w481 w485]
                          tunnel: w478 -> [w482 w488]
                          tunnel: [w480 w487] -> w465
                          tunnel: [w479 w484] -> w477
                          tunnel: w470 -> [w483 w486]
                          frame False {
                            n267 = Subtract(x=w483, y=w482) -> (x-y=w479:dbl)
                            n268 = Greater Or Equal?(x=w479, y=w481) -> (x >= y?=w480:bool)
                          }
                          frame True {
                            n269 = Add(x=w486, y=w488) -> (x+y=w484:dbl)
                            n270 = Less Or Equal?(x=w484, y=w485) -> (x <= y?=w487:bool)
                          }
                        }
                        n271 = Quotient & Remainder(x=w470, y=w469) -> (x-y*floor(x/y)=w471:dbl, floor(x/y)=w468:dbl)
                        n272 = Not Equal To 0?(x=w471) -> (x != 0?=w466:bool)
                        n273 = Equal To 0?(x=w468) -> (x = 0?=w467:bool)
                        n274 = Or(x=w466, y=w467) -> ()  [unwired: 1 out]
                        n275 = case shown="True" w465 {
                          tunnel: w477 -> [_ w499]
                          tunnel: [TRUE FALSE] -> w476
                          tunnel: [FALSE w500] -> w475
                          tunnel: w470 -> [_ w497]
                          tunnel: w473 -> [_ w496]
                          tunnel: w472 -> [_ w495]
                          frame False {
                          }
                          frame True {
                            n276 = local read "step [V]"() -> (w493:dbl)
                            n277 = call "SupplyRamp.vi"("error in"=w496, "Requested Voltage"=w499, "Step Size"=w493, "Step Delay"=100, "Supply IN"=w495, "Starting Voltage"=w497) -> ("error out"=w491:errorcluster, "Compliance exceeded"=w500:bool, "Current Voltage"=w494:dbl)  [unwired: 2 in, 1 out]
                            n278 = case shown="No Error" w491 {
                              tunnel: w494 -> [w502 _]
                              frame No Error {
                                n279 = local write "Current Volts:"(w502) -> ()
                              }
                              frame Error {
                              }
                            }
                            n280 = property on="Bias On/Off:" class="Bool (strict)"("Blinking"=w500) -> ()  [unwired: 2 in, 2 out]
                            n281 = local write "STATUS 1"("Incrementing volts.") -> ()
                          }
                        }
                      }
                    }
                  }
                  frame True {
                    w503 = FALSE
                  }
                }
              }
            }
            n282 = case shown="True" w261 {
              frame False {
              }
              frame True {
                n283 = property on="Bias On/Off:" class="Bool (strict)"("Blinking"=TRUE) -> ()  [unwired: 2 in, 2 out]
              }
            }
            n284 = Build Array(w263, w261, "abort", w262) -> (w267:bool[])
            n285 = Or Array Elements(Boolean array=w267) -> (logical OR=w273:bool)
            n286 = Not(x=w273) -> (.not. x?=w272:bool)
          }
        }
        frame True {
          w505 = FALSE
          # "compliance was exceeded when first voltage applied."
          # "Flag compliance as reason for end of run"
          n287 = local write "STATUS 1"("Run aborted - compliance exceeded.") -> ()
          n288 = Build Array(w505, TRUE, w505, w505) -> (w506:bool[])
        }
      }
      n289 = Search 1D Array(1D array=w250, element=TRUE) -> (index of element=w248:i32)  [unwired: 1 in]
      n290 = Increment(x=w248) -> (x+1=w247:i32)
      n291 = case shown="..0" w247 {
        tunnel: ["" "Run ended normally" "Compliance exceeded" "Run aborted - by user" "Run aborted - Ilimit exceeded"] -> w242
        frame ..0 {
        }
        frame 1 {
        }
        frame 2 {
          # "Determine reason for end of run."
        }
        frame 3 {
        }
        frame 4.. {
        }
      }
      n292 = global read "QC_RunInformation.vi" "Run info"() -> (w246:T6)
      n293 = Bundle By Name(cluster=w246, "End of Run comment:"=w242) -> (w241:T6)
      n294 = Concatenate Strings(w242, "\r\n", "RAMPING DOWN VOLTS") -> (w245:string)
      n295 = global write "QC_RunInformation.vi" "Run info"(w241) -> ()
      n296 = local write "STATUS 1"(w245) -> ()
    }
    frame #4 {
      # "Ramp down and switch off supply"
      n297 = stacked-sequence {
        frame #0 {
          # "Tie up loose ends. Set volts to zero and switch to standby"
          # "Ramp down volts now"
          n298 = global read "QC_MeasurementSetup.vi" "Cis Measurement Parameters"() -> (w517:T8)
          n299 = Unbundle By Name(w517) -> ("Supply"=w514:refnum<class "SupplyControl.lvclass">, "Ramp down steps [V]"=w516:dbl, "Ramp down Interval [s]"=w515:i32, "Switching"=w510:refnum<class "Switching.lvclass">, "Matrix used?"=w511:bool)
          n300 = local read "Current Volts:"() -> (w522:dbl)
          n301 = Multiply(x=w515, y=1000) -> (x*y=w519:i32)
          n302 = call "SupplyRamp.vi"("Requested Voltage"=0.0, "Step Size"=w516, "Step Delay"=w519, "Supply IN"=w514, "Starting Voltage"=w522) -> ("error out"=w513:errorcluster, "Supply OUT"=w512:refnum<class "SupplyControl.lvclass">, "Current Voltage"=w520:dbl)  [unwired: 3 in, 1 out]
          n303 = call-dynamic "Supply_Stby.vi"("error in (no error)"=w513, "SupplyControl in"=w512) -> ("error out"=w509:errorcluster)  [unwired: 8 in, 1 out]
          n304 = local write "Current Volts:"(w520) -> ()
          n305 = case shown="True" w511 {
            tunnel: w510 -> [_ w527]
            tunnel: w509 -> [_ w526]
            frame False {
            }
            frame True {
              n306 = call-dynamic "MatrixSwitch.vi"("error in (no error)"=w526, "Action"=T4."Reset", "Switching in"=w527) -> ("error out"=w523:errorcluster, "Switching out"=w524:refnum<class "Switching.lvclass">)  [unwired: 6 in, 1 out]
              n307 = call-dynamic "Close.vi"("error in (no error)"=w523, "Switching in"=w524) -> ()  [unwired: 8 in, 2 out]
            }
          }
        }
        frame #1 {
          w532 = 0
          n308 = local write "Bias On/Off:"(FALSE ("Visible")) -> ()
          n309 = local write "Current Volts:"(0.0 ("Current Volts:")) -> ()
          n310 = property on="abort" class="Bool (strict)"("DisabledEnum"=2) -> ()  [unwired: 2 in, 2 out]
          n311 = property on="Quit & Save" class="Bool"("DisabledEnum"=w532) -> ()  [unwired: 2 in, 2 out]
          n312 = property on="quit (no save)" class="Bool"("DisabledEnum"=w532) -> ()  [unwired: 2 in, 2 out]
          n313 = local write "STATUS 1"("Run finished. \nSave data?" ("STATUS 1")) -> ()
        }
        frame #2 {
          n314 = Current VI's Path() -> (path=w534:path)
          n315 = call "SaveJPEG.vi"("Test"="Cis", "File Path Control"=w534) -> ()  [unwired: 1 in, 2 out]
        }
      }
    }
    frame #5 {
      # "Loop and await decision on whether to save or junk data"
      # "Display and save data"
      n316 = local read "Cscale"() -> (w544:enum16{"1/C^2 [1/nF^2]", "nF", "pF"})
      n317 = local read "Scales"() -> (w545:T1)
      n318 = while {
        shift-left: w544 -> [w595]
        shift-right: [w594] -> _
        shift-left: w545 -> [w597]
        shift-right: [w596] -> _
        tunnel: ["Quit & Save"] -> w547
        tunnel: ["quit (no save)"] -> w546
        stop <- w592 continue-if-true
        n319 = local read "Scales"() -> (w596:T1)
        n320 = local read "Cscale"() -> (w594:enum16{"1/C^2 [1/nF^2]", "nF", "pF"})
        n321 = Not Equal?(x=w597, y=w596) -> (x != y?=w590:bool)
        n322 = Not Equal?(x=w595, y=w594) -> (x != y?=w589:bool)
        n323 = case shown="True" w590 {
          tunnel: w596 -> [_ w624]
          frame False {
          }
          frame True {
            n324 = case shown="\"Log - log\".." w624 {
              tunnel: [w625 1 0 w630] -> w623
              tunnel: [w625 0 1 w630] -> w622
              frame .."Lin - Lin" {
                w625 = 0
              }
              frame "Log - Lin" {
              }
              frame "Lin - Log" {
              }
              frame "Log - log".. {
                w630 = 1
              }
            }
            n325 = property on="Cgraph" class="WFGraph (strict)"("X Scale.Mapping Mode"=w623) -> ()  [unwired: 2 in, 2 out]
            n326 = property on="Cgraph" class="WFGraph (strict)"("Y Scale.Mapping Mode"=w622, "YScale.Minimum"=w622) -> ()  [unwired: 2 in, 2 out]
          }
        }
        n327 = case shown="True" w589 {
          tunnel: w594 -> [_ w602]
          frame False {
          }
          frame True {
            n328 = property on="Cgraph" class="WFGraph (strict)"() -> ("YScale.Mapping Mode"=w605:u8)  [unwired: 2 in, 2 out]
            n329 = global read "QC_MeasurementSetup.vi" "Cis Measurement Parameters"() -> (w604:T8)
            n330 = property on="Cgraph" class="WFGraph (strict)"("YScale.Minimum"=w605) -> ()  [unwired: 2 in, 2 out]
            n331 = Unbundle By Name(w604) -> ("Initial Voltage [V]"=w607:dbl, "Step Size [V]"=w609:dbl, "Number Of Steps"=w606:u32)
            n332 = call "CisData.vi"("Action"=T3."Read Array", "Array No."=u32 1 ("Action")) -> ("Array OUT"=w598:dbl[])  [unwired: 3 in, 1 out]
            n333 = Absolute Value(x=w609) -> (abs(x)=w608:dbl)
            n334 = Array Subset(array=w598, index=0, length=w606) -> (w610:dbl[])
            n335 = Absolute Value(x=w610) -> (abs(x)=w603:dbl[])
            n336 = case shown="..\"1/C^2 [1/nF^2]\"" w602 {
              tunnel: [w615 w618 w621] -> w601
              tunnel: w603 -> [w613 w620 w621]
              frame .."1/C^2 [1/nF^2]" {
                n337 = Array Size(array=w613) -> (size(s)=w614:i32)
                n338 = for {
                  N: w614 -> [_]
                  tunnel: w613 -> [w617] mode=indexing
                  tunnel: [w616] -> w615 mode=indexing
                  n339 = formula code="y=1000000./(x*x);"("x"=w617) -> ("y"=w616:dbl)
                }
              }
              frame "nF" {
                n340 = Divide(x=w620, y=1000.0) -> (x/y=w618:dbl[])
              }
              frame "pF".. {
              }
            }
            n341 = Bundle("Initial Voltage [V]"=w607, w608, w601) -> (w611:cluster{"Initial Voltage [V]":dbl, dbl, dbl[]})  [unwired: 1 in]
            n342 = local write "Cgraph"(w611) -> ()
          }
        }
        n343 = Not Or(1:"quit (no save)", 2:"Quit & Save") -> (0:w592:bool)
      }
      n344 = global read "QC_MeasurementSetup.vi" "Cis Measurement Parameters"() -> (w543:T8)
      n345 = Unbundle By Name(w543) -> ("Temperature Readout"=w542:enum16{"Read Arduino", "Enter manually"}, "Arduino"=w536:refnum<class "ArduinoControl.lvclass">)
      n346 = case shown="\"Read Arduino\"" w542 {
        tunnel: w536 -> [_ w588]
        frame "Enter manually", Default {
        }
        frame "Read Arduino" {
          n347 = call "ArduinoClose.vi"("ArduinoControl in"=w588) -> ()  [unwired: 9 in, 2 out]
        }
      }
      n348 = case shown="True" w546 {
        tunnel: [FALSE w632] -> w548
        frame False {
        }
        frame True {
          n349 = Two Button Dialog(message="Are you sure you don't want to save the data?", 1:"Quit" ("F button name (\"Cancel\")"), 2:"Save data" ("T button name (\"OK\")")) -> (T button?=w632:bool)
        }
      }
      n350 = Or(x=w547, y=w548) -> (x .or. y?=w541:bool)
      n351 = flat-sequence {
        tunnel: w541 -> [w550]
        tunnel: [w550] -> w537
        tunnel: [TRUE] -> w535
        frame #0 {
          n352 = global read "QC_MeasurementSetup.vi" "Cis Measurement Parameters"() -> (w560:T8)
          n353 = Unbundle By Name(w560) -> ("C_is Limit [pF/cm]"=w553:dbl, "Number Of Steps"=w555:u32)
          n354 = call "ScanFeedback.vi"("measurement type"=T5."Cis") -> ("Cis @300V [pF/cm]"=w551:dbl)  [unwired: 4 in, 4 out]
          n355 = case shown="True" w550 {
            tunnel: ["" w587] -> w561
            tunnel: [_ w570] -> w559
            tunnel: w555 -> [_ w567]
            frame False {
            }
            frame True {
              w568 = T3."Read Array" ("Action")
              n356 = local write "STATUS 1"("Saving Data ...") -> ()
              n357 = call "CisData.vi"("Action"=w568, "Array No."=u32 2 ("Action")) -> ("Array OUT"=w565:dbl[])  [unwired: 3 in, 1 out]
              n358 = Multiply(x=w565, y=0.001) -> (x*y=w564:dbl[])
              n359 = call "CisData.vi"("Action"=w568, "Array No."=u32 0 ("Action")) -> ("Array OUT"=w577:dbl[])  [unwired: 3 in, 1 out]
              n360 = call "CisData.vi"("Action"=w568, "Array No."=u32 1 ("Action")) -> ("Array OUT"=w576:dbl[])  [unwired: 3 in, 1 out]
              n361 = Build Array(w577, w576, w564) -> (w575:dbl[][])
              n362 = call "CisData.vi"("Action"=w568, "Array No."=u32 4 ("Action")) -> ("Array OUT"=w583:dbl[])  [unwired: 3 in, 1 out]
              n363 = call "CisData.vi"("Action"=w568, "Array No."=u32 3 ("Action")) -> ("Array OUT"=w582:dbl[])  [unwired: 3 in, 1 out]
              n364 = call <vilib>:"Std Deviation and Variance.vi"("X"=w583) -> ("mean"=w571:dbl)  [unwired: 1 in, 2 out]
              n365 = call <vilib>:"Std Deviation and Variance.vi"("X"=w582) -> ("mean"=w572:dbl)  [unwired: 1 in, 2 out]
              n366 = Transpose 2D Array(2D array=w575) -> (transposed array=w574:dbl[][])
              n367 = call "SaveDataFile.vi"("Data Array"=w574, "Temperature"=w572, "Humidity"=w571, "no. of arrays"=3, "Actual array lengths"=w567, "Array Titles"="Voltage[V] Capacitance[pF] Resistance[kOhm]", "Strip Segment"="", "Arrays format"="%010.2f") -> ("Path + Filename OUT"=w587:string, "Error Out"=w570:errorcluster)  [unwired: 4 in, 2 out]
            }
          }
          n368 = Absolute Value(x=w551) -> (abs(x)=w554:dbl)
          n369 = Absolute Value(x=w553) -> (abs(x)=w552:dbl)
          n370 = Less Or Equal?(x=w554, y=w552) -> (x <= y?=w556:bool)
          n371 = call "WriteLogFile.vi"("Automatic warning"="", "Data File"=w561, "Error In"=w559, "DUT passed?"=w556, "Value TechSpec criteria"=w551, "Files saved?"=w550) -> ()  [unwired: 5 in, 1 out]
        }
      }
      n372 = Select(t="Run finished.\nData saved." ("STATUS 1"), s=w537, f="Run finished.\nData not saved." ("STATUS 1")) -> (s? t:f=w540:string)
      n373 = local write "STATUS 1"(w540) -> ()
      "Done!" <- w535
    }
  }
